vi "Bead Tracking Find beads.vi"(5 "Match Pattern Setup Data":string, 6 "Minimum Match Score":sgl=800.0 min=0 max=1000 format="%.2f", 7 "Search Rectangle":T4, 8 "error in (no error)":errorcluster, 9 "Bead Tracking Mode":T2, 10 "Template":T3, 11 "Image":T3) -> (0 "error out":errorcluster, 1 "Number of Matches":i32, 2 "Raw matches":T1(array[cluster]) {"Bounding Box"."y" format="%.2f"; "Bounding Box"."x" format="%.2f"; "Position"."y" format="%.2f"; "Position"."x" format="%.2f"; "Score" format="%.2f"; "Scale" format="%.2f"; "Angle" format="%.2f"}, 3 "Image out":T3)   [LabVIEW 2011]
doc: "This is a small wrapper around \"IMAQ Match Pattern 2\" (in NI_Vision_Development_Module.lvlib)"
uses:
  <vilib>/vision/Image Controls.llb/IMAQ Image.ctl
  Bead Tracking Mode.ctl
  <vilib>/vision/NI_Vision_Development_Module.lvlib
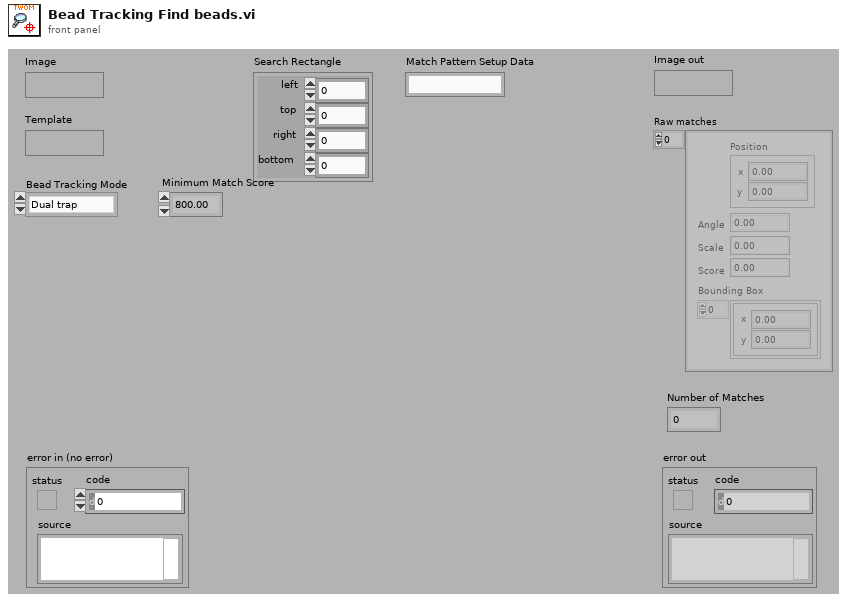
[diagram p1: front panel]
types:
  T1 = cluster{"Position":cluster{"x":sgl, "y":sgl}, "Angle":sgl, "Scale":sgl, "Score":sgl, "Bounding Box":cluster{"x":sgl, "y":sgl}[]}[]
  T2 = typedef "Bead Tracking Mode.ctl" = enum16{"Dual trap", "Q-trap =", "Q-trap ||", "Q-trap X", "Q-trap +", "Dual trap oO", "Single trap", "None"}
  T3 = typedef "IMAQ Image.ctl" = refnum<image>
  T4 = cluster{"left":i16, "top":i16, "right":i16, "bottom":i16}
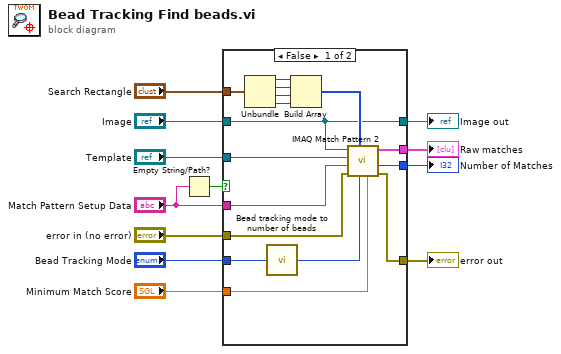
[diagram p0: block diagram]
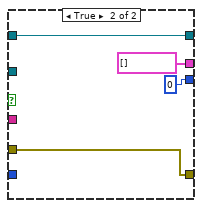
[diagram p2: hidden frame]
diagram:
  n1 = Empty String/Path?(string/path="Match Pattern Setup Data") -> (empty?=w2:bool)
  n2 = case shown="False" w2 {
    tunnel: "Image" -> [w13 w32]
    tunnel: "Template" -> [w28 _]
    tunnel: "Search Rectangle" -> [w27 _]
    tunnel: "error in (no error)" -> [w21 w29]
    tunnel: [w20 w29] -> w8
    tunnel: [w19 0 ("Number of Matches")] -> w7
    tunnel: "Minimum Match Score" -> [w18 _]
    tunnel: "Bead Tracking Mode" -> [w17 _]
    tunnel: [w15 T1 [] ("Matches")] -> w4
    tunnel: "Match Pattern Setup Data" -> [w14 _]
    tunnel: [w13 w32] -> w1
    frame False {
      n3 = Unbundle(w27) -> ("left"=w26:i16, "top"=w25:i16, "right"=w24:i16, "bottom"=w23:i16)
      n4 = call "Bead tracking mode to number of beads.vi"("Bead Tracking Mode"=w17) -> ("Number of beads"=w16:i32)
      n5 = Build Array(w26, w25, w24, w23) -> (w22:i16[])
      n6 = call "IMAQ Match Pattern 2"("Minimum Match Score"=w18, "Number of Matches Requested"=w16, "Optional Rectangle"=w22, "error in (no error)"=w21, "Match Pattern Setup Data"=w14, "Template Image"=w28, "Image"=w13) -> ("error out"=w20:errorcluster, "Number of Matches"=w19:i32, "Matches"=w15:T1)  [unwired: 2 out]
    }
    frame True {
    }
  }
  "error out" <- w8
  "Number of Matches" <- w7
  "Image out" <- w1
  "Raw matches" <- w4
